vi "Open Account.vi"() -> (0 "error out":errorcluster, 3 "Account info":T1)   [LabVIEW 2012]
uses:
  Account Info.ctl
  Stop.vi
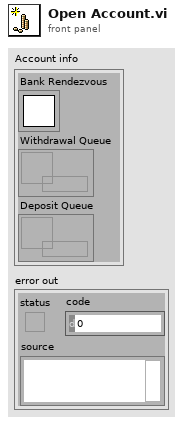
[diagram p1: front panel]
types:
  T1 = typedef "Account Info.ctl" = cluster{"Bank Rendezvous":T2, "Withdrawal Queue":refnum<queue>, "Deposit Queue":refnum<queue>}
  T2 = typedef "Rendezvous RefNum" = refnum<k1>
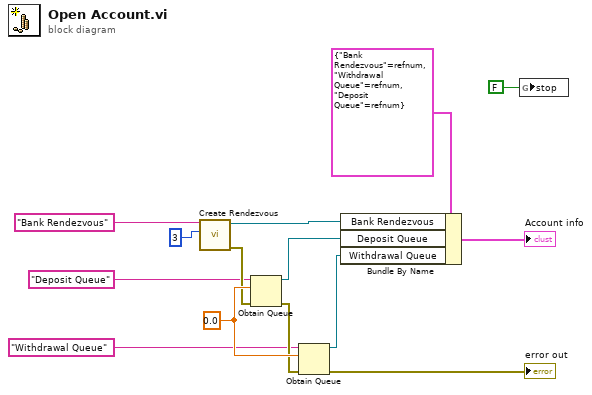
[diagram p0: block diagram]
diagram:
  w13 = 0.0
  n1 = call <vilib>:"Create Rendezvous.vi"("size (2)"=3, "name (unnamed)"="Bank Rendezvous") -> ("error out"=w12:errorcluster, "rendezvous"=w14:T2)  [unwired: 3 in, 1 out]
  n2 = Obtain Queue(name (unnamed)="Deposit Queue", element data type=w13, error in (no error)=w12) -> (queue out=w10:refnum<queue>, error out=w11:errorcluster)  [unwired: 2 in, 1 out]
  n3 = Obtain Queue(name (unnamed)="Withdrawal Queue", element data type=w13, error in (no error)=w11) -> (queue out=w9:refnum<queue>, error out=→"error out":errorcluster)  [unwired: 2 in, 1 out]
  n4 = Bundle By Name(cluster=T1 {"Bank Rendezvous"=refnum, "Withdrawal Queue"=refnum, "Deposit Queue"=refnum}, "Bank Rendezvous"=w14, "Deposit Queue"=w10, "Withdrawal Queue"=w9) -> (→"Account info":T1)
  n5 = global write "Stop.vi" "stop"(FALSE ("stop")) -> ()
